vi "SetVoltage.vi"(8 "error in":errorcluster, 11 "Voltage":dbl=200.0 format="%.2f") -> (0 "error out":errorcluster)   [LabVIEW 2010]
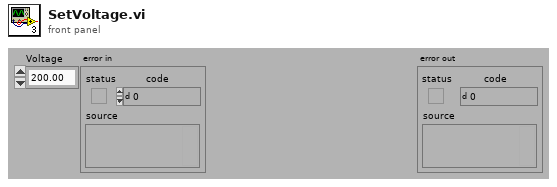
[diagram p1: front panel]
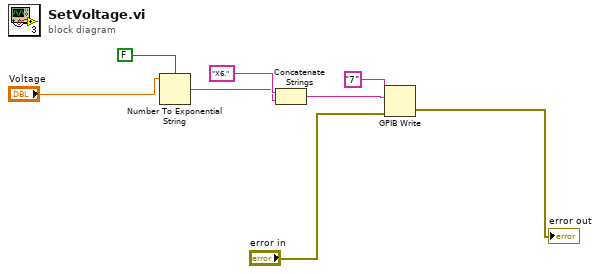
[diagram p0: block diagram]
diagram:
  n1 = Number To Exponential String(number="Voltage", 1:FALSE) -> (E-format string=w4:string)  [unwired: 2 in]
  n2 = Concatenate Strings("X6.", w4) -> (w3:string)
  n3 = GPIB Write(0:"7", 1:w3, 3:"error in") -> (6:→"error out":errorcluster)  [unwired: 2 in, 1 out]
